vi "Test FTDI SPI SYS Read.vi"() -> ()   [LabVIEW 2018]
uses:
  PROJEKT/NIKO/Labview/Niko V4/FTDI SPI/Ctl/Sub Addr.ctl
panel:
  in  "nCS":u8 max=4 step=1
  out "Out Reg A Bin":bool[](array[boolean])
  out "Out Reg B Bin":bool[](array[boolean])
  in  "Addr":T1 items=["Addr-0", "Addr-1", "Addr-2", "Addr-3", "Addr-4", "Addr-5", "Addr-6", "Addr-7"]
  out "error out":errorcluster
  out "Ini Status":bool
  in  "config":T2={"ClockRate"=50000, "LatencyTimer"=10, "configOptions 24-31"=0, "configOptions 16-23"=0, "configOptions 8-15"=0, "configOptions 0-7"=32, "Pin"=0, "reserved"=0} {"configOptions 24-31" format="%x"; "configOptions 16-23" format="%x"; "configOptions 8-15" format="%x"; "configOptions 0-7" format="%x"}
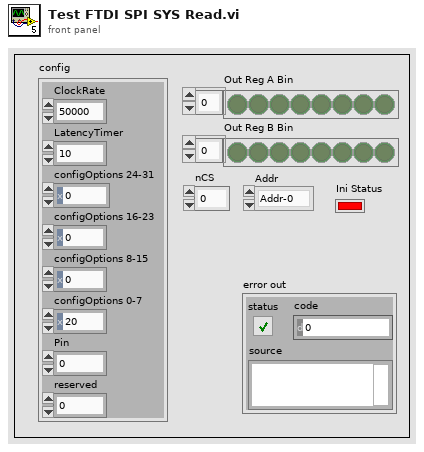
[diagram p1: front panel]
types:
  T1 = typedef "Sub Addr.ctl" = u16
  T2 = cluster{"ClockRate":u32, "LatencyTimer":u8, "configOptions 24-31":i8, "configOptions 16-23":i8, "configOptions 8-15":i8, "configOptions 0-7":u32, "Pin":u32, "reserved":u16}
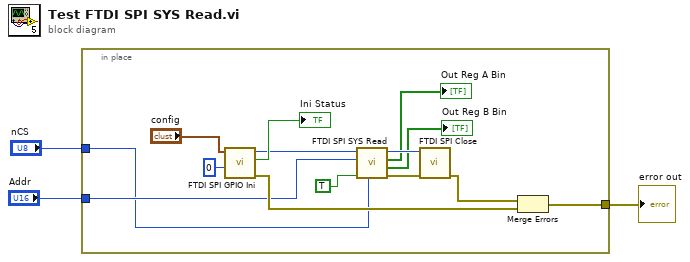
[diagram p0: block diagram]
diagram:
  n1 = in-place {
    in-place-border: [w15] -> w3
    in-place-border: "Addr" -> [w10]
    in-place-border: "nCS" -> [w4]
    n2 = call "FTDI SPI GPIO Ini.vi"("Channel Nmb"=u8 0 ("FTDI Dev Nmb"), "config"="config") -> ("error out"=w14:errorcluster, "Ini Status"=→"Ini Status":bool, "handle out"=w12:u32)  [unwired: 5 in, 2 out]
    n3 = call "FTDI SPI SYS Read.vi"("nCS"=w4, "Use Extra"=TRUE, "Addr"=w10, "Handler In"=w12) -> ("error out"=w8:errorcluster, "Out Reg B Bin"=→"Out Reg B Bin":bool[], "Out Reg A Bin"=→"Out Reg A Bin":bool[], "Handler Out"=w9:u32)  [unwired: 2 in, 2 out]
    n4 = call "FTDI SPI Close.vi"("error in (no error)"=w8, "Handler In"=w9) -> ("error out"=w13:errorcluster)  [unwired: 9 in]
    n5 = Merge Errors(w13, w14) -> (w15:errorcluster)
  }
  "error out" <- w3
